vi "Update Commit Complete.vi"(6 "Review Complete?":bool, 8 "error in":errorcluster, 10 "Commit ID":i32, 11 "Peer Review in":refnum<class "Peer Review.lvclass">) -> (0 "error out":errorcluster, 3 "Peer Review out":refnum<class "Peer Review.lvclass">)   [LabVIEW 2020, in "Peer Review.lvclass"]
uses:
  Peer Review.lvclass
  Peer Review.lvclass/Peer Review.ctl
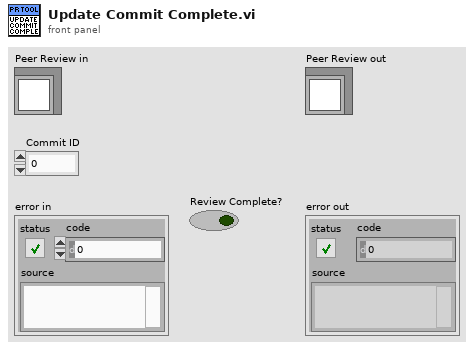
[diagram p1: front panel]
types:
  T1 = typedef "Peer Review.lvclass/File Info.ctl" = cluster{"File ID":i32, "Commit ID":i32, "Reviewed Hash":string, "Relative Path":string, "File Path":path, "File Checksum":string, "State":T2, "FP Changes":i32, "BD Changes":i32, "FP Bounds Error":dbl, "BD Bounds Error":dbl, "Lines Added":i32, "Lines Removed":i32, "Analysis Passes":i32, "Analysis Fails":i32, "Attribute Changes":i32, "Reentrancy State":string, "Cyclomatic Complexity":i32, "Node Count":i32, "Revision Number":u32, "LabVIEW Version":string, "Description":string, "Master Path":path, "Master Checksum":string, "VI Type":T3, "LabVIEW File":bool, "Review Complete":bool, "File Ref":refnum<vi>}
  T2 = typedef "Peer Review.lvclass/File State.ctl" = enum16{"Interrogation Needed", "Modified", "Deleted", "Added", "Matches Previous", "No Changes", "Moved"}
  T3 = typedef "Peer Review.lvclass/VI Type.ctl" = enum32{"invalid VI type", "Standard VI", "Control VI", "Global VI", "Polymorphic VI", "Configuration VI", "SubSystem", "Facade VI", "Method VI", "Statechart Diagram VI"}
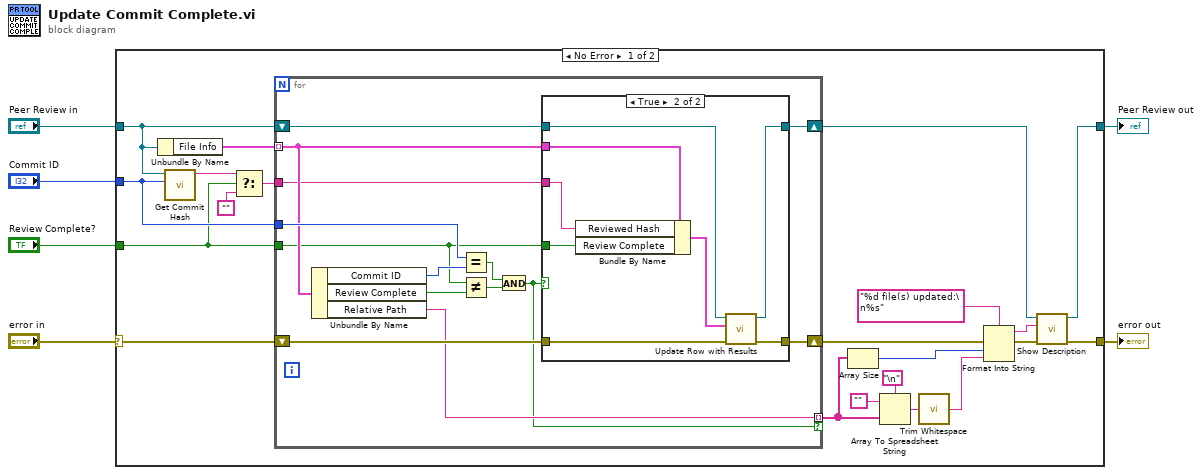
[diagram p0: block diagram]
diagram:
  n1 = case shown="No Error" "error in" {
    selector: "error in" -> [w25 w52]
    tunnel: "Commit ID" -> [w27 _]
    tunnel: "Peer Review in" -> [w26 w53]
    tunnel: [w14 w52] -> w3
    tunnel: [w12 w53] -> w2
    tunnel: "Review Complete?" -> [w10 _]
    frame No Error {
      n2 = Unbundle By Name(w26) -> ("File Info"=w24:T1[])
      n3 = call "Get Commit Hash.vi"("Commit ID"=w27, "Peer Review"=w26) -> ("Hash"=w9:string)  [unwired: 9 in]
      n4 = Select(t=w9, s=w10, f="" ("Empty String Constant")) -> (s? t:f=w8:string)
      n5 = for {
        tunnel: w24 -> [w39] mode=indexing
        tunnel: w27 -> [w41]
        shift-right: [w36] -> w15
        shift-left: w25 -> [w38]
        shift-right: [w35] -> w13
        shift-left: w26 -> [w37]
        tunnel: w8 -> [w34]
        tunnel: w10 -> [w30]
        tunnel: [w29] -> w11 mode=indexing if=w28
        n6 = Unbundle By Name(w39) -> ("Commit ID"=w40:i32, "Review Complete"=w33:bool, "Relative Path"=w29:string)
        n7 = Equal?(x=w41, y=w40) -> (x = y?=w31:bool)
        n8 = Not Equal?(x=w30, y=w33) -> (x != y?=w32:bool)
        n9 = And(x=w31, y=w32) -> (x .and. y?=w28:bool)
        n10 = case shown="True" w28 {
          tunnel: w39 -> [_ w51]
          tunnel: w38 -> [w42 w50]
          tunnel: w37 -> [w43 w49]
          tunnel: [w42 w47] -> w36
          tunnel: [w43 w46] -> w35
          tunnel: w34 -> [_ w45]
          tunnel: w30 -> [_ w44]
          frame False {
          }
          frame True {
            n11 = Bundle By Name(cluster=w51, "Reviewed Hash"=w45, "Review Complete"=w44) -> (w48:T1)
            n12 = call "Update Row with Results.vi"("error in"=w50, "File Info"=w48, "Peer Review in"=w49) -> ("error out"=w47:errorcluster, "Peer Review out"=w46:refnum<class "Peer Review.lvclass">)  [unwired: 7 in]
          }
        }
      }
      n13 = Array Size(array=w11) -> (size(s)=w21:i32)
      n14 = Array To Spreadsheet String(delimiter (Tab)="\n" ("Line Feed Constant"), array=w11, 3:"" ("Empty String Constant")) -> (spreadsheet string=w20:string)
      n15 = call <vilib>:"Trim Whitespace.vi"("string"=w20) -> ("trimmed string"=w19:string)  [unwired: 1 in]
      n16 = Format Into String(format string="%d file(s) updated:\n%s", error in=w15, w21, w19) -> (resulting string=w16:string, error out=w17:errorcluster)  [unwired: 1 in]
      n17 = call "Show Description.vi"("error in"=w17, "Description"=w16, "Peer Review in"=w13) -> ("error out"=w14:errorcluster, "Peer Review out"=w12:refnum<class "Peer Review.lvclass">)  [unwired: 7 in]
    }
    frame Error {
    }
  }
  "Peer Review out" <- w2
  "error out" <- w3
